vi "class to JSON.vi"   [LabVIEW 2018, in "LV-Julia_ZMQ-Roundtrip_lib.lvlib" / "testclass.lvclass"]
uses:
  testclass.lvclass
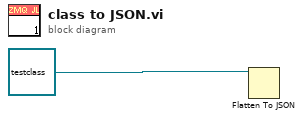
[diagram p0: block diagram]
diagram:
  n1 = Flatten To JSON(anything=refnum<class "testclass.lvclass"> refnum ("LV-Julia_ZMQ-Roundtrip_lib.lvlib:testclass.lvclass")) -> ()  [unwired: 2 in, 2 out]
